vi "Transfer Function V-F.vi"() -> ()   [LabVIEW 2017]
uses:
  <vilib>/DAQmx/read.llb/DAQmx Read (Analog DBL 1Chan 1Samp).vi
  <vilib>/DAQmx/create/channels.llb/DAQmx Create Channel (AI-Voltage-Basic).vi
  <vilib>/DAQmx/miscellaneous.llb/DAQmx Fill In Error Info.vi
panel:
  out "Force measure":dbl(graph)
  out "Output Voltage Force Sensor":dbl(graph)
  in  "stop":bool
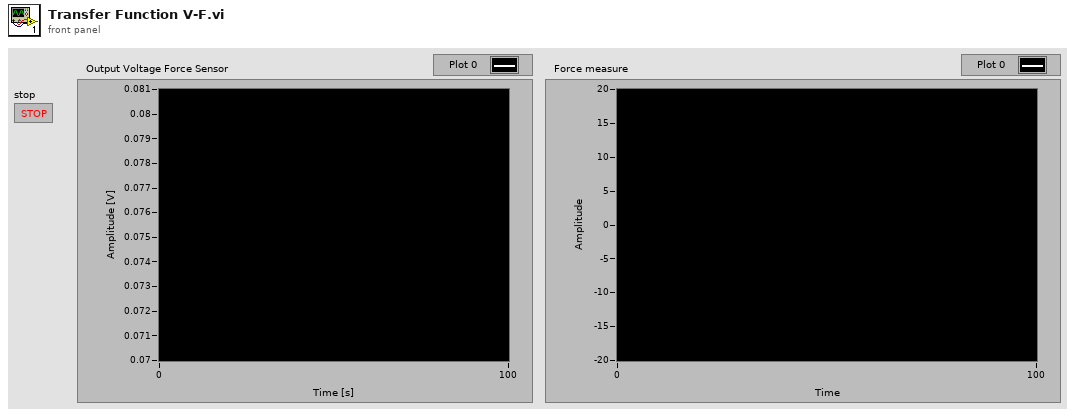
[diagram p1: front panel]
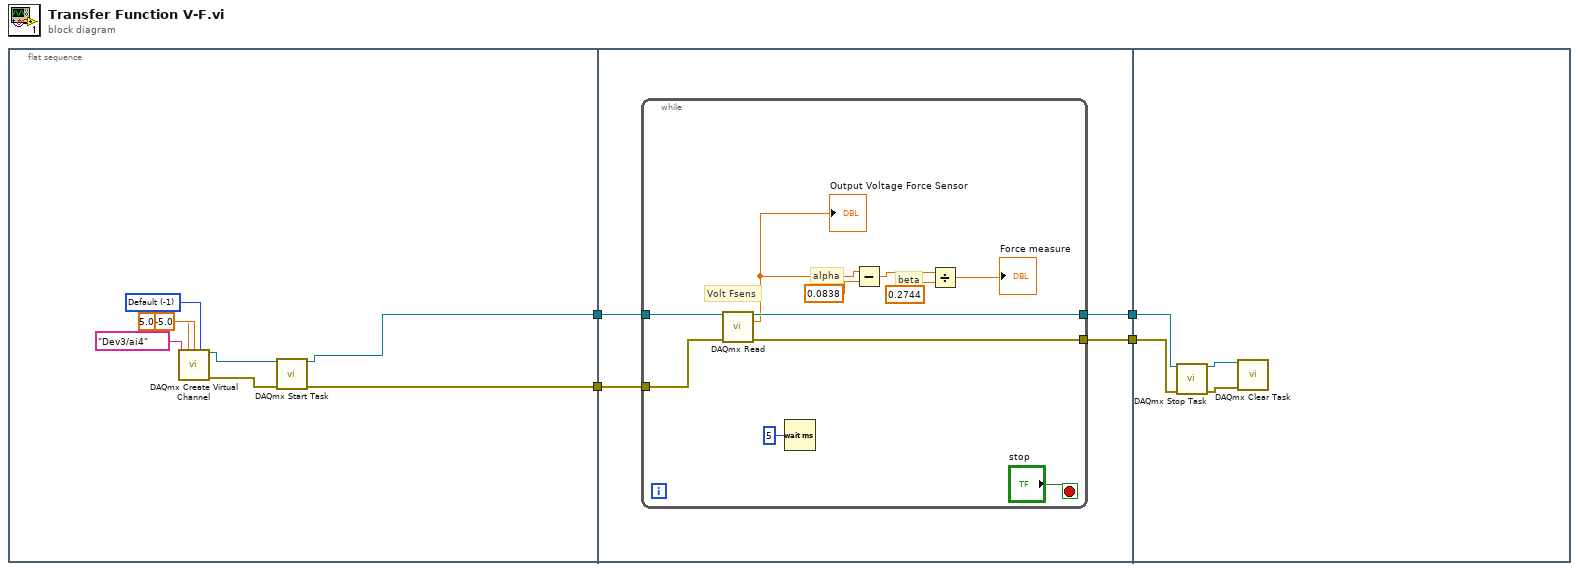
[diagram p0: block diagram]
diagram:
  n1 = flat-sequence {
    tunnel: [w10] -> w4
    tunnel: [w8] -> w2
    tunnel: w4 -> [w16]
    tunnel: [w15] -> w3
    tunnel: w2 -> [w14]
    tunnel: [w13] -> w1
    tunnel: w3 -> [w31]
    tunnel: w1 -> [w29]
    frame #0 {
      w5 = -1 items=["Default"=-1, "RSE"=10083, "NRSE"=10078, "Differential"=10106, "Pseudodifferential"=12529] ("input terminal configuration")
      n2 = call-poly <vilib>:"DAQmx Create Virtual Channel.vi"("maximum value"=5.0, "minimum value"=-5.0, "input terminal configuration"=w5, "physical channels"=tag "Dev3/ai4") -> ("task out"=w11:refnum<k21>, "error out"=w9:errorcluster)  [unwired: 10 in]
      n3 = call <vilib>:"DAQmx Start Task.vi"("task/channels in"=w11, "error in"=w9) -> ("task out"=w10:refnum<k21>, "error out"=w8:errorcluster)  [unwired: 12 in]
    }
    frame #1 {
      n4 = while {
        tunnel: w16 -> [w27]
        tunnel: [w26] -> w15
        tunnel: w14 -> [w25]
        tunnel: [w24] -> w13
        stop <- "stop" stop-if-true
        # "Volt Fsens"
        # "beta"
        # "alpha"
        n5 = call-poly <vilib>:"DAQmx Read.vi"("task/channels in"=w27, "error in"=w25) -> ("task out"=w26:refnum<k21>, "data"=w21:dbl, "error out"=w24:errorcluster)  [unwired: 11 in]
        "Output Voltage Force Sensor" <- w21
        n6 = Wait (ms)(milliseconds to wait=u32 5) -> ()  [unwired: 1 out]
        n7 = Subtract(x=w21, y=0.0838) -> (x-y=w20:dbl)
        n8 = Divide(x=w20, y=0.2744) -> (x/y=→"Force measure":dbl)
      }
    }
    frame #2 {
      n9 = call <vilib>:"DAQmx Stop Task.vi"("task/channels in"=w31, "error in"=w29) -> ("task out"=w30:refnum<k21>, "error out"=w28:errorcluster)  [unwired: 12 in]
      n10 = call <vilib>:"DAQmx Clear Task.vi"("task in"=w30, "error in"=w28) -> ()  [unwired: 13 in, 1 out]
    }
  }
